vi "Climb Loop.vi"() -> (1 "Unpin Power":dbl, 2 "Pull Power":dbl, 3 "PTO Engaged?":bool)   [LabVIEW 2015]
uses:
  Common Code/Climb Auto State.ctl
  Robot Global Data.vi
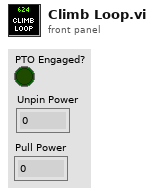
[diagram p1: front panel]
types:
  T1 = typedef "Dashboard Control Data.ctl" = cluster{"Shooter Presets":T2, "Encoder Control":T4, "Steer PID output":cluster{"output high":dbl, "output low":dbl}, " Steer PID gains":cluster{"proportional gain (Kc)":dbl, "integral time (Ti, min)":dbl, "derivative time (Td, min)":dbl}, "Drivetrain Settings":T5, "Vision Packet":T6, "Dashboard Drivetrain Command":T7, "Info/Command Cluster":T9, "Ball Vision Packet":T10, "Intake Presets":T12, "Intake Encoder Control":T14, "Climb Presets":T15, "Ultrasonic Limit":dbl, "Roll Limit":dbl, "Pitch Limit":dbl, "Goal Output Range":cluster{"output high":dbl, "output low":dbl}}
  T2 = typedef "Shooter Presets.ctl" = cluster{"Batter Shot":T3, "Deep Middle Shot":T3, "Manual Shot":T3, "Left Ticks Per Rotation":dbl, "Right Ticks Per Rotation":dbl, "Low Bar Shot":T3, "Shooter RPM Tolerance":dbl, "IIR Filter Power":dbl, "Trigger Power":dbl, "Fire from Load Delay":i32, "Angle Pot M":dbl, "Angle Pot B":dbl, "Shooter Length":dbl, "String Pot Dist":dbl, "Angle PID gains":cluster{"proportional gain (Kc)":dbl, "integral time (Ti, min)":dbl, "derivative time (Td, min)":dbl}, "Angle Motor Output":cluster{"output high":dbl, "output low":dbl}, "Shooter Angle Tolerance":dbl, "Vision Shoot x^2":dbl, "Vision Shoot x":dbl, "Dist from Axis Cam to Pivot":dbl, "High Goal Center Height":dbl, "Feed Forward Max Accel":dbl, "Feed Forward Kv":dbl, "Backwards Trigger":dbl, "Shot Finish Delay (ms)":dbl, "Angle Max Current":dbl, "Angle Current Trip Time":dbl, "Shooter Intake Angle":dbl, "Vision Shoot c":dbl, "Reset?":bool, "Servo Release Delay":dbl, "Servo Idle Angle":i32, "Servo Hold Angle":i32, "Angle Pot x^2":dbl, "Angle Pot x":dbl, "Angle Pot c":dbl, "Ignore Angle?":bool}
  T3 = typedef "Shot Presets.ctl" = cluster{"Left Wheel RPM":dbl, "Right Wheel RPM":dbl, "Angle":dbl}
  T4 = typedef "Encoder Control.ctl" = cluster{"Right Tick Constant":dbl, "Left Tick Constant":dbl, "Reset?":bool, "Y Dist":cluster{"PID gains":cluster{"proportional gain (Kc)":dbl, "integral time (Ti, min)":dbl, "derivative time (Td, min)":dbl}}, "Y Stop Thresh":dbl, "Y Stop Speed":dbl}
  T5 = typedef "Drivetrain Settings.ctl" = cluster{"Gyro Tolerance":dbl, "Throttle Ramp (ms)":dbl, "Angular rate compensation":bool, "Throttle to Rate Scale":dbl, "Rate compensation gain":dbl, "Kv":dbl, "Ka":dbl, "Feed Forward P":dbl, "Feed Forward D":dbl, "Goal Vision PID gains":cluster{"proportional gain (Kc)":dbl, "integral time (Ti, min)":dbl, "derivative time (Td, min)":dbl}, "Goal Detection Window":dbl}
  T6 = typedef "Goal Vision Packet.ctl" = cluster{"Distance":dbl, "Center X":dbl, "Center Y":dbl, "Found Target?":bool}
  T7 = typedef "Dashboard Drivetrain Command.ctl" = cluster{"Drivetrain Vision":T8}
  T8 = typedef "Drivetrain Vision.ctl" = cluster{"Goal Window":dbl, "Ball Window":dbl}
  T9 = typedef "Ball Tracking Command Cluster.ctl" = cluster{"Distance to Ball":dbl, "Desired Angle":dbl, "Command":enum16{"Turn to Ball", "Turn to Angle", "Get Distance"}, "Pixels from Center":dbl}
  T10 = typedef "Ball Vision Packet.ctl" = cluster{"Ball Detected?":bool, "Distance to Ball":dbl, "Desired Angle":dbl, "Pixels from Center":dbl, "Tracking mode":T11}
  T11 = typedef "Tracking Mode.ctl" = enum16{"Turn to Ball", "Turn to Angle"}
  T12 = typedef "Intake Presets.ctl" = cluster{"Intake Speed":dbl, "Outake Speed":dbl, "Low Height":dbl, "Half Height":dbl, "Full Height":dbl, "Angle Speed":dbl, "Fast Angle":dbl, "Encoder Scale":dbl, "Load Height":dbl, "Output Range":T13, "Rotation Power Max/Min":dbl, "MaxCurrent":dbl, "Intake Trip Time":dbl, "Idle Height":dbl, "Max Height":dbl, "Reset Encoders?":bool, "PID gains":cluster{"proportional gain (Kc)":dbl, "integral time (Ti, min)":dbl, "derivative time (Td, min)":dbl}}
  T13 = typedef "Drivetrain Output Range.ctl" = cluster{"output high":dbl, "output low":dbl}
  T14 = typedef "IntakeEcoderControl.ctl" = cluster{"Arm Tick Constant":dbl, "Reset?":bool, "Y Dist":cluster{"PID gains":cluster{"proportional gain (Kc)":dbl, "integral time (Ti, min)":dbl, "derivative time (Td, min)":dbl}}, "Y Stop Thresh":dbl, "Y Stop Speed":dbl}
  T15 = typedef "Climb Presets.ctl" = cluster{"Pull Power":dbl, "Unpin Power":dbl, "Time to Hold":dbl}
  T16 = typedef "Climb Command Cluster.ctl" = cluster{"Climb Mode":T17, "Hold?":bool, "Manual State":T18}
  T17 = typedef "Climb Mode.ctl" = enum16{"Auto", "Manual"}
  T18 = typedef "Climb Manual State.ctl" = cluster{"Release":bool, " PTO Engage":bool}
  T19 = typedef "Encoder Values Super Cluster.ctl" = cluster{"Left Encoder":T20, "Right Encoder":T20}
  T20 = typedef "Encoder Values.ctl" = cluster{"Distance":dbl, "Speed":dbl, "Ticks":dbl}
  T21 = typedef "Climb Auto State.ctl" = enum16{"Reach up", "Hold on", "Pull up"}
  T22 = typedef "Climb Status Cluster.ctl" = cluster{"Pull Power":dbl, "Unpin Power":dbl, "PTO Engaged?":bool, "Pull Height":dbl}
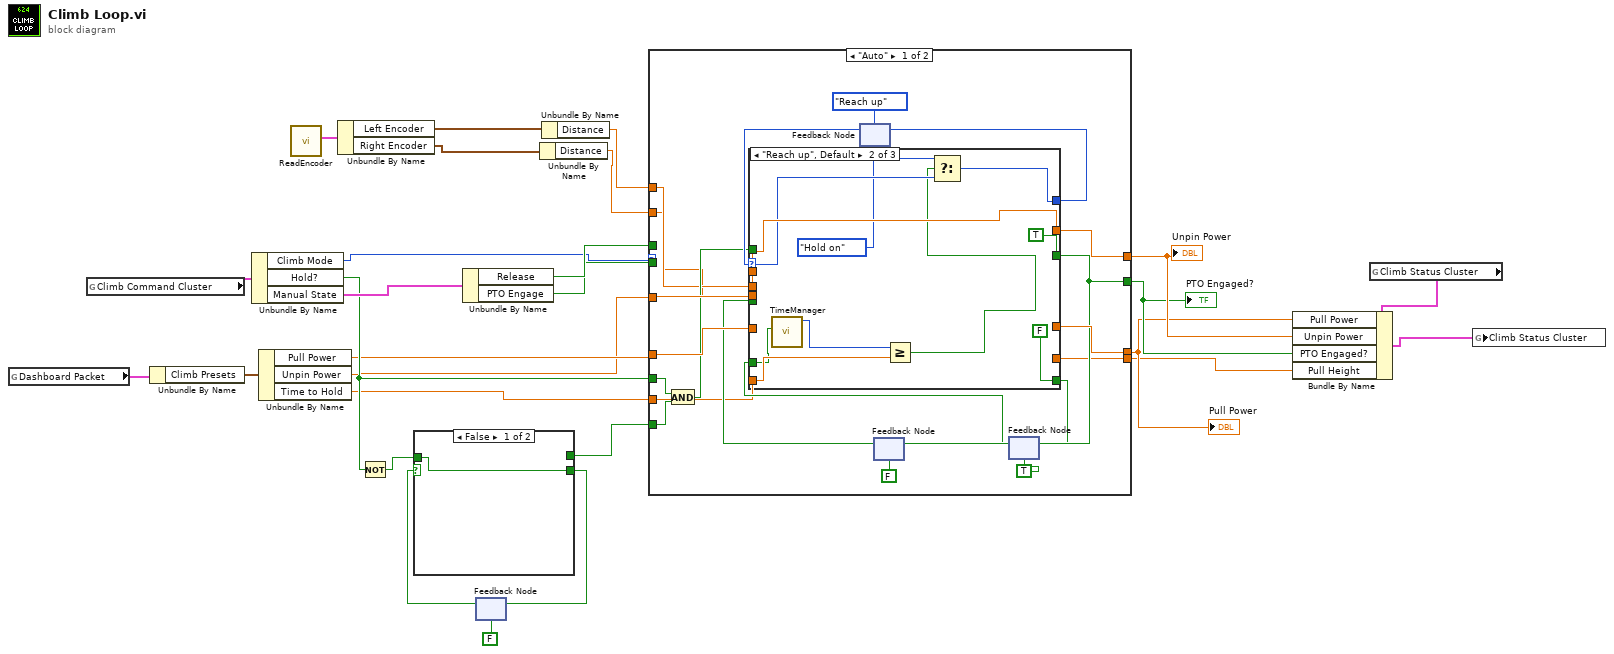
[diagram p0: block diagram]
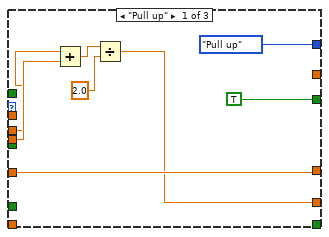
[diagram p2: hidden frame]
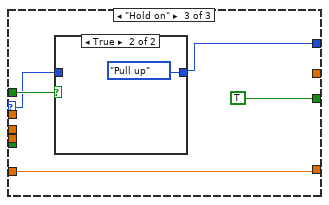
[diagram p3: hidden frame]
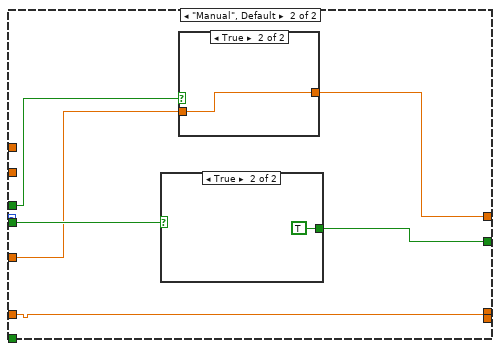
[diagram p5: hidden frame]
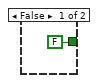
[diagram p6: hidden frame]
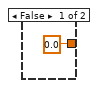
[diagram p7: hidden frame]
diagram:
  n1 = global read "Robot Global Data.vi" "Dashboard Packet"() -> (w12:T1)
  n2 = global read "Robot Global Data.vi" "Climb Command Cluster"() -> (w18:T16)
  n3 = Unbundle By Name(w12) -> ("Climb Presets"=w13:T15)
  n4 = Unbundle By Name(w18) -> ("Climb Mode"=w20:T17, "Hold?"=w17:bool, "Manual State"=w19:T18)
  n5 = Unbundle By Name(w13) -> ("Pull Power"=w16:dbl, "Unpin Power"=w15:dbl, "Time to Hold"=w14:dbl)
  n6 = call "ReadEncoder.vi"() -> ("Quick Use Cluster"=w2:T19)  [unwired: 11 in]
  n7 = Unbundle By Name(w2) -> ("Left Encoder"=w4:T20, "Right Encoder"=w3:T20)
  n8 = Not(x=w17) -> (.not. x?=w23:bool)
  n9 = Unbundle By Name(w19) -> ("Release"=w22:bool, "PTO Engage"=w21:bool)
  n10 = feedback #1(FALSE) -> (w24:bool)
  n11 = case shown="False" w24 {
    selector: w24 -> [_ w29]
    tunnel: [w28 w29] -> w26
    tunnel: [_ w29] -> w25
    tunnel: w23 -> [w28 _]
    frame False {
    }
    frame True {
    }
  }
  n12 = feedback-in #1(w26) -> ()
  n13 = Unbundle By Name(w3) -> ("Distance"=w1:dbl)
  n14 = Unbundle By Name(w4) -> ("Distance"=w5:dbl)
  n15 = case shown="\"Auto\"" w20 {
    tunnel: w16 -> [w49 w75]
    tunnel: [w48 w75] -> w9
    tunnel: [w46 w77] -> w10
    tunnel: w22 -> [_ w80]
    tunnel: w25 -> [w38 _]
    tunnel: [w42 w79] -> w11
    tunnel: w21 -> [_ w78]
    tunnel: w15 -> [w43 w76]
    tunnel: w17 -> [w39 _]
    tunnel: w14 -> [w33 _]
    tunnel: [w32 _] -> w8
    tunnel: w5 -> [w31 _]
    tunnel: w1 -> [w30 _]
    frame "Auto" {
      n16 = And(x=w39, y=w38) -> (x .and. y?=w37:bool)
      n17 = feedback #2(Climb_Auto_State."Reach up" ("Auto State")) -> (w47:T21)
      n18 = feedback #3(FALSE ("PTO Engage")) -> (w44:bool)
      n19 = feedback #4(TRUE) -> (w36:bool)
      n20 = case shown="\"Reach up\", Default" w47 {
        selector: w47 -> [_ w65 w70]
        tunnel: w49 -> [w56 _ w68]
        tunnel: [w56 _ w68] -> w48
        tunnel: [Climb_Auto_State."Pull up" ("Auto State") w64 w69] -> w40
        tunnel: [TRUE ("PTO Engage") TRUE ("PTO Engage") TRUE ("PTO Engage")] -> w46
        tunnel: w44 -> [_ _ _]
        tunnel: w37 -> [_ _ w71]
        tunnel: w43 -> [_ w67 _]
        tunnel: [_ w67 _] -> w42
        tunnel: w33 -> [_ w62 _]
        tunnel: w36 -> [_ w60 _]
        tunnel: [_ FALSE _] -> w35
        tunnel: [w54 _ _] -> w32
        tunnel: w30 -> [w52 _ _]
        tunnel: w31 -> [w51 _ _]
        frame "Pull up" {
          n21 = Add(x=w51, y=w52) -> (x+y=w53:dbl)
          n22 = Divide(x=w53, y=2.0) -> (x/y=w54:dbl)
        }
        frame "Reach up", Default {
          n23 = call "TimeManager.vi"("Reset?"=w60) -> ("Time Since Reset"=w61:u32)  [unwired: 9 in, 1 out]
          n24 = Greater Or Equal?(x=w61, y=w62) -> (x >= y?=w63:bool)
          n25 = Select(t=Climb_Auto_State."Hold on" ("Auto State"), s=w63, f=w65) -> (s? t:f=w64:T21)
        }
        frame "Hold on" {
          n26 = case shown="True" w71 {
            tunnel: [w73 Climb_Auto_State."Pull up" ("Auto State")] -> w69
            tunnel: w70 -> [w73 _]
            frame False {
            }
            frame True {
            }
          }
        }
      }
      n27 = feedback-in #2(w40) -> ()
      n28 = feedback-in #3(w46) -> ()
      n29 = feedback-in #4(w35) -> ()
    }
    frame "Manual", Default {
      n30 = case shown="True" w78 {
        tunnel: [FALSE TRUE] -> w77
        frame False {
        }
        frame True {
        }
      }
      n31 = case shown="True" w80 {
        tunnel: [0.0 w84] -> w79
        tunnel: w76 -> [_ w84]
        frame False {
        }
        frame True {
        }
      }
    }
  }
  "Pull Power" <- w9
  "PTO Engaged?" <- w10
  "Unpin Power" <- w11
  n32 = global read "Robot Global Data.vi" "Climb Status Cluster"() -> (w6:T22)
  n33 = Bundle By Name(cluster=w6, "Pull Power"=w9, "Unpin Power"=w11, "PTO Engaged?"=w10, "Pull Height"=w8) -> (w7:T22)
  n34 = global write "Robot Global Data.vi" "Climb Status Cluster"(w7) -> ()
